vi "CH1603_Init COM.vi"(8 "error in (no error)":errorcluster, 10 "Baud Rate(19200)":u32(ring)=19200 items=["300"=300, "600"=600, "1200"=1200, "2400"=2400, "4800"=4800, "9600"=9600, "19200"=19200, "115200"=115200], 11 "MyIndex":u8) -> (0 "error out":errorcluster, 2 "status":bool, 3 "VISA resource name out":refnum<visa-resource-name>)   [LabVIEW 2015]
doc: "Initial the CH1603B device serial port,the default band rate is 19200. must be use this VI before call other control or read VI."
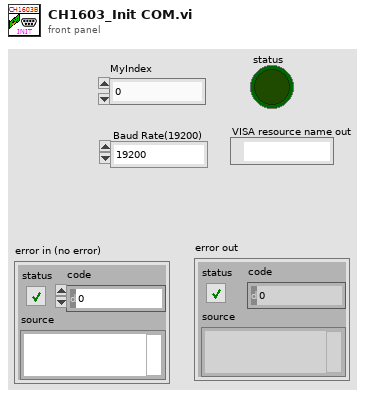
[diagram p1: front panel]
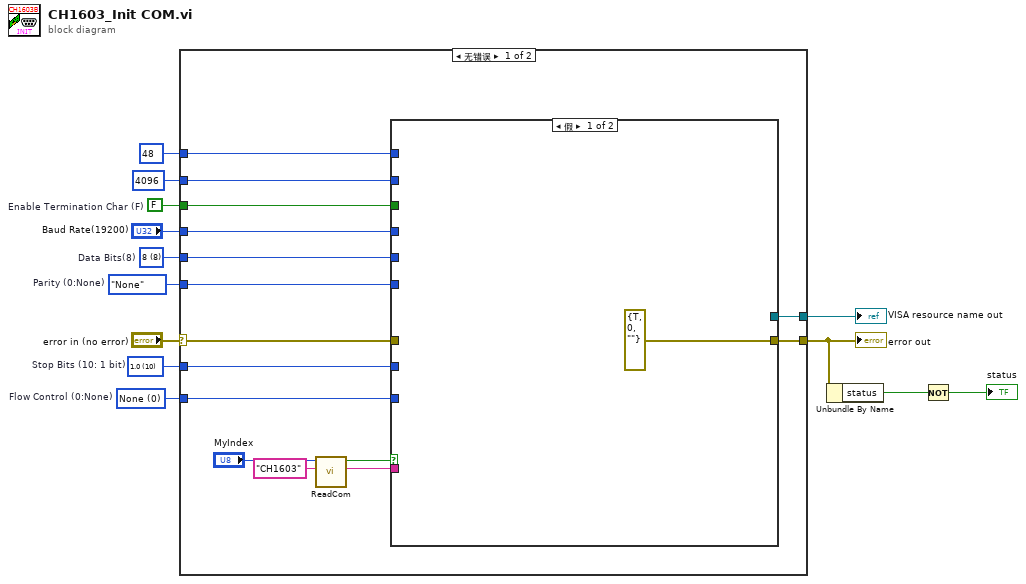
[diagram p0: block diagram]
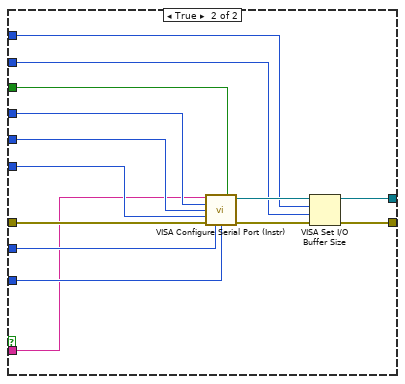
[diagram p2: hidden frame]
diagram:
  w4 = u16 0 items=["None", "XON/XOFF", "RTS/CTS", "XON/XOFF & RTS/CTS", "DTR/DSR", "XON/XOFF & DTR/DSR"]  # Flow Control (0:None)
  w5 = FALSE  # Enable Termination Char (F)
  w9 = u16 10 items=["1.0"=10, "1.5"=15, "2.0"=20]  # Stop Bits (10: 1 bit)
  w6 = enum16{"None", "Odd", "Even", "Mark", "Space"}."None"  # Parity (0:None)
  w7 = u16 8 items=["7"=7, "8"=8]  # Data Bits(8)
  n1 = case shown="无错误" "error in (no error)" {
    selector: "error in (no error)" -> [w28 w44]
    tunnel: [w27 w44] -> w3
    tunnel: [w26 _] -> w12
    tunnel: u32 4096 ("Buffer Size(4096)") -> [w25 _]
    tunnel: u16 48 ("mask (16)") -> [w24 _]
    tunnel: w9 -> [w23 _]
    tunnel: "Baud Rate(19200)" -> [w22 _]
    tunnel: w7 -> [w21 _]
    tunnel: w6 -> [w20 _]
    tunnel: w5 -> [w19 _]
    tunnel: w4 -> [w18 _]
    frame No Error {
      n2 = call "ReadCom.vi"("仪器名称"="CH1603", "MyIndex"="MyIndex") -> ("COM"=w14:string, "OK?"=w15:bool)  [unwired: 7 in, 1 out]
      n3 = case shown="假" w15 {
        tunnel: w28 -> [_ w43]
        tunnel: [errorcluster {"status"=TRUE, "code"=0, "source"=""} ("error out") w40] -> w27
        tunnel: [_ w39] -> w26
        tunnel: w25 -> [_ w38]
        tunnel: w24 -> [_ w37]
        tunnel: w23 -> [_ w36]
        tunnel: w22 -> [_ w35]
        tunnel: w21 -> [_ w34]
        tunnel: w20 -> [_ w33]
        tunnel: w19 -> [_ w32]
        tunnel: w18 -> [_ w31]
        tunnel: w14 -> [_ w30]
        frame False {
        }
        frame True {
          n4 = call <vilib>:"VISA Configure Serial Port (Instr).vi"("VISA resource name"=w30, "Enable Termination\nChar (T)"=w32, "baud rate (9600)"=w35, "data bits (8)"=w34, "parity (0:none)"=w33, "error in (no error)"=w43, "stop bits (10: 1 bit)"=w36, "flow control (0:none)"=w31) -> ("VISA resource name out"=w41:refnum<visa-resource-name>, "error out"=w42:errorcluster)  [unwired: 6 in]
          n5 = VISA Set I/O Buffer Size(VISA resource name=w41, mask (16)=w37, size (4096)=w38, error in (no error)=w42) -> (VISA resource name out=w39:refnum<visa-resource-name>, error out=w40:errorcluster)
        }
      }
    }
    frame Error {
    }
  }
  "VISA resource name out" <- w12
  "error out" <- w3
  n6 = Unbundle By Name(w3) -> ("status"=w2:bool)
  n7 = Not(x=w2) -> (.not. x?=→"status":bool)
